vi "Self Test.vi"(8 "error in":errorcluster, 11 "69X_79X in":refnum<class "6972A.lvclass">) -> (0 "error out":errorcluster, 3 "69X_79X out":refnum<class "6972A.lvclass">)   [LabVIEW 2019, in "6972A.lvlib" / "6972A.lvclass"]
uses:
  Library/6972A.lvclass
  builds/Instruments/PowerSupply.lvlibp/Library/PowerSupply.lvclass
  <instrlib>/Agilent N6900 N7900 Series/Agilent N6900 N7900 Series.lvlib
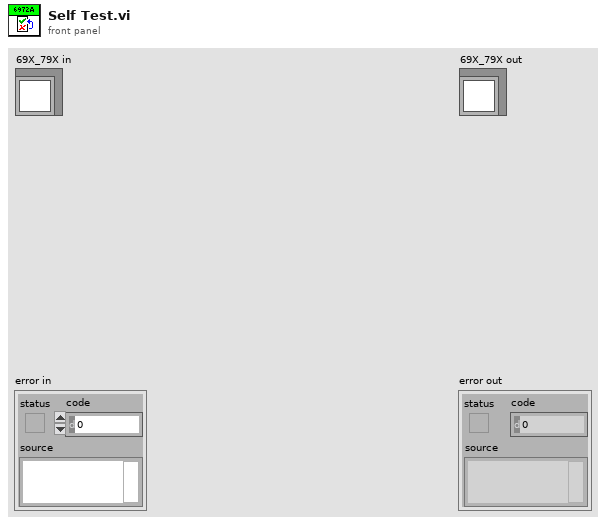
[diagram p1: front panel]
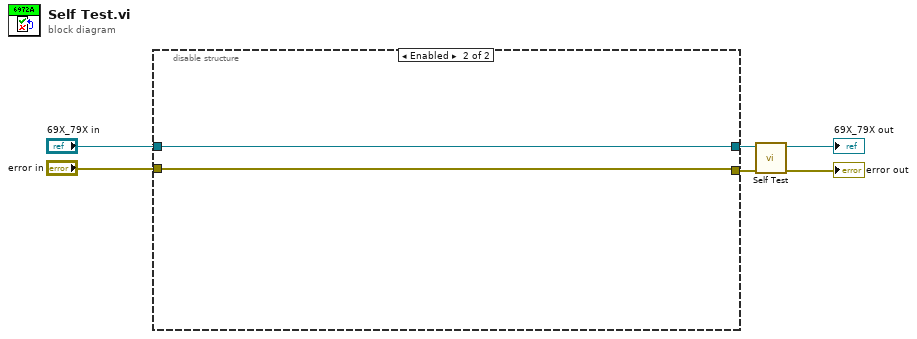
[diagram p0: block diagram]
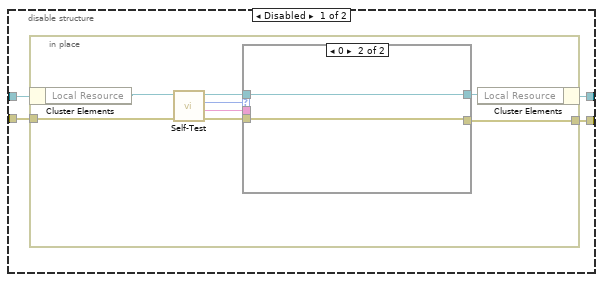
[diagram p2: hidden frame]
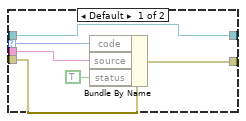
[diagram p3: hidden frame]
diagram:
  n1 = disable-structure shown="Enabled" {
    disable-tunnel: "69X_79X in" -> [w10 w28]
    disable-tunnel: "error in" -> [w9 w27]
    disable-tunnel: [w8 w28] -> w4
    disable-tunnel: [w7 w27] -> w2
    frame Disabled {
      n2 = in-place {
        in-place-border: w9 -> [w17]
        in-place-border: [w11] -> w7
        n3 = in-place-cluster #1(w10) -> ("Local Resource"=w18:refnum<visa-resource-name>)
        n4 = call <instrlib>:"Self-Test.vi"("error in (no error)"=w17, "VISA resource name"=w18) -> ("error out"=w14:errorcluster, "Self-Test Result Message"=w13:string, "Self-Test Result Code"=w16:i32, "VISA resource name out"=w15:refnum<visa-resource-name>)  [unwired: 6 in]
        n5 = case shown="0" w16 {
          selector: w16 -> [w23 _]
          tunnel: w15 -> [w19 w25]
          tunnel: w14 -> [w24 w26]
          tunnel: w13 -> [w22 _]
          tunnel: [w20 w26] -> w11
          tunnel: [w19 w25] -> w12
          frame Default {
            n6 = Bundle By Name(cluster=w24, "code"=w23, "source"=w22, "status"=TRUE) -> (w20:errorcluster)
          }
          frame 0 {
          }
        }
        n7 = in-place-cluster #1("Local Resource"=w12) -> (w8:refnum<class "6972A.lvclass">)
      }
    }
    frame Enabled {
    }
  }
  n8 = call-parent "Self Test.vi"("error in"=w2, "Instruments in"=w4) -> ("error out"=→"error out":errorcluster, "Instruments out"=→"69X_79X out":refnum<class "6972A.lvclass">)  [unwired: 8 in]
